vi "CohortReadElectrode.vi"(8 "error in (no error)":errorcluster, 10 "Index":u8, 11 "Cohort in":refnum<class "Cohort.lvclass">) -> (0 "error out":errorcluster, 2 "Electrode out":refnum<class "Electrode.lvclass">, 3 "Cohort out":refnum<class "Cohort.lvclass">)   [LabVIEW 2012, in "Cohort.lvclass"]
uses:
  Cohort.lvclass
  Electrode.lvclass
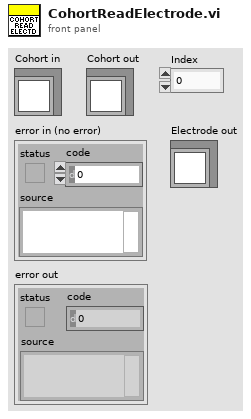
[diagram p1: front panel]
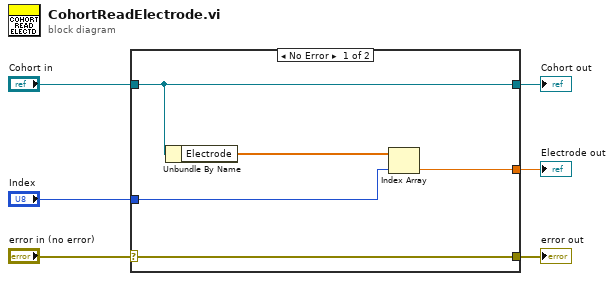
[diagram p0: block diagram]
diagram:
  n1 = case shown="No Error" "error in (no error)" {
    selector: "error in (no error)" -> [w11 w12]
    tunnel: [w11 w12] -> w5
    tunnel: [w10 w13] -> w3
    tunnel: "Cohort in" -> [w10 w13]
    tunnel: [w8 _] -> w2
    tunnel: "Index" -> [w7 _]
    frame No Error {
      n2 = Unbundle By Name(w10) -> ("Electrode"=w9:sgl[])
      n3 = Index Array(array=w9, index=w7) -> (element=w8:sgl)
    }
    frame Error {
    }
  }
  "error out" <- w5
  "Cohort out" <- w3
  "Electrode out" <- w2
